vi "LSX Magazin Seated.vi"(8 "error in (no error)":errorcluster, 9 "status":i32, 10 "maga":i32, 11 "lLSID":i32) -> (0 "error out":errorcluster, 1 "status out":i32, 3 "function return":i32)   [LabVIEW 2018, in "Tango.lvlib"]
doc: "TANGOAPI int TANGOCALL LSX_MagazinSeated (int lLSID, int maga, int *status);"
uses:
  Tango.lvlib
  SubVIs/Tango_DLL.dll
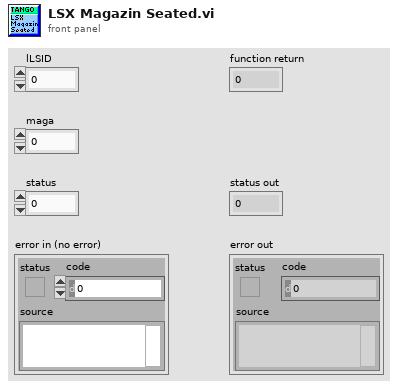
[diagram p1: front panel]
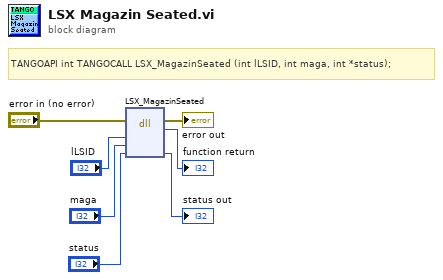
[diagram p0: block diagram]
diagram:
  # "TANGOAPI int TANGOCALL LSX_MagazinSeated (int lLSID, int maga, int *status);"
  n1 = dll-call lib="C:/Users/Familie/Documents/LabviewIX81/lib/TANGO Stage/SubVIs/Tango_DLL.*" fn="LSX_MagazinSeated"(error in="error in (no error)", "lLSID"="lLSID", "maga"="maga", "status"="status") -> (error out=→"error out":errorcluster, →"function return":i32, "status"=→"status out":i32)  [unwired: 4 in, 1 out]
